vi "createsamplinginfo.vi"(5 "Integer Degree of Nonlinearity (RF) (N) ( y(t) = x^1(t) + ...  + x^N(t) )":i32=1, 6 "Low Side / High Side tuning":bool, 7 "Integer Degree of Nonlinearity (LO) (N) ( y(t) = x^1(t) + ...  + x^N(t) )":i32=2, 8 "Duration (Seconds)":dbl=1e-05, 9 "RF Passband Bandwidth (Hz)":dbl=100000000.0 format="%#_6p", 10 "Intermediate Frequency":dbl=600000000.0 format="%#_6p", 11 "RF Carrier Frequency":dbl=1000000000.0 format="%#_6p") -> (1 "Number of Samples":dbl, 2 "Sampling Frequency":dbl, 3 "LO Frequency":dbl)   [LabVIEW 2009]
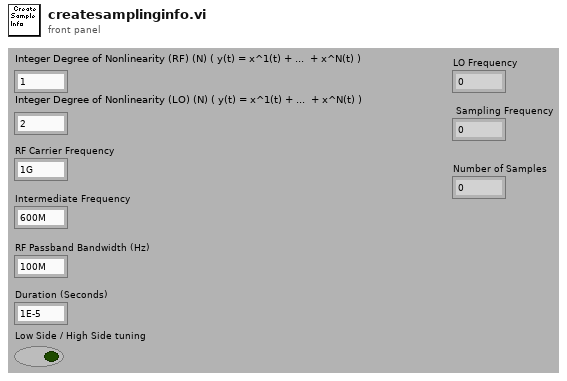
[diagram p1: front panel]
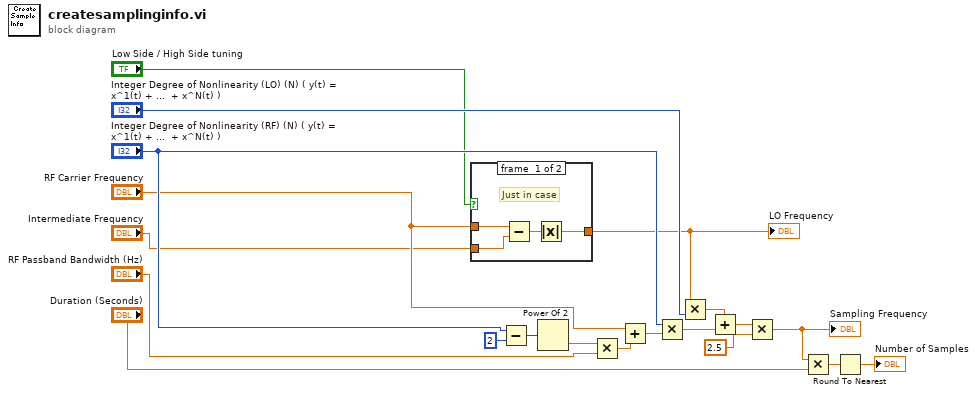
[diagram p0: block diagram]
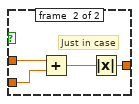
[diagram p2: hidden frame]
diagram:
  n1 = case shown="True" "Low Side / High Side tuning" {
    tunnel: "RF Carrier Frequency" -> [w24 w28]
    tunnel: "Intermediate Frequency" -> [w23 w27]
    tunnel: [w21 w25] -> w1
    frame #0 {
      # "Just in case"
      n2 = Subtract(x=w24, y=w23) -> (x-y=w22:dbl)
      n3 = Absolute Value(x=w22) -> (abs(x)=w21:dbl)
    }
    frame #1 {
      # "Just in case"
      n4 = Add(x=w28, y=w27) -> (x+y=w26:dbl)
      n5 = Absolute Value(x=w26) -> (abs(x)=w25:dbl)
    }
  }
  "LO Frequency" <- w1
  n6 = Subtract(x="Integer Degree of Nonlinearity (RF) (N) ( y(t) = x^1(t) + ...  + x^N(t) )", y=2) -> (x-y=w10:i32)
  n7 = Power Of 2(x=w10) -> (2^x=w11:dbl)
  n8 = Multiply(x=w11, y="RF Passband Bandwidth (Hz)") -> (x*y=w12:dbl)
  n9 = Add(x="RF Carrier Frequency", y=w12) -> (x+y=w13:dbl)
  n10 = Multiply(x="Integer Degree of Nonlinearity (RF) (N) ( y(t) = x^1(t) + ...  + x^N(t) )", y=w13) -> (x*y=w14:dbl)
  n11 = Multiply(x=w1, y="Integer Degree of Nonlinearity (LO) (N) ( y(t) = x^1(t) + ...  + x^N(t) )") -> (x*y=w16:dbl)
  n12 = Add(x=w16, y=w14) -> (x+y=w17:dbl)
  n13 = Multiply(x=w17, y=2.5) -> (x*y=w18:dbl)
  "Sampling Frequency" <- w18
  n14 = Multiply(x=w18, y="Duration (Seconds)") -> (x*y=w19:dbl)
  n15 = Round To Nearest(number=w19) -> (nearest integer value=→"Number of Samples":dbl)
